vi "Launch Standard Configuration Editor.vi"   [LabVIEW 2013]
uses:
  Standard Editor/Standard Editor.lvlib
types:
  T1 = enum32{"Invalid", "Standard", "Closed", "Hidden", "Minimized", "Maximized"}
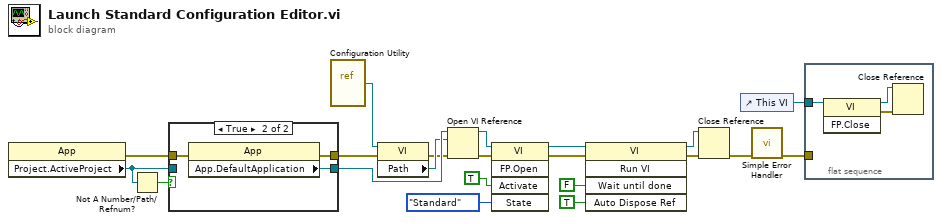
[diagram p0: block diagram]
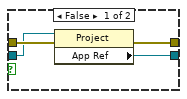
[diagram p2: hidden frame]
diagram:
  n1 = property class="App"() -> (error out=w20:errorcluster, "Project.ActiveProject"=w11:refnum<vi>)  [unwired: 2 in, 1 out]
  n2 = Not A Number/Path/Refnum?(number/path/refnum=w11) -> (NaN/Path/Refnum?=w10:bool)
  n3 = case shown="True" w10 {
    tunnel: w20 -> [w25 w28]
    tunnel: [w24 w26] -> w19
    tunnel: [w23 w27] -> w8
    tunnel: w11 -> [w22 _]
    frame False {
      n4 = property class="Project"(reference=w22, error in=w25) -> (error out=w23:errorcluster, "App Ref"=w24:refnum<vi>)  [unwired: 1 out]
    }
    frame True {
      n5 = property class="App"(error in=w28) -> (error out=w27:errorcluster, "App.DefaultApplication"=w26:refnum<vi>)  [unwired: 1 in, 1 out]
    }
  }
  n6 = vi-ref "Configuration Utility.vi"() -> (w21:refnum<vi>)
  n7 = property class="VI"(reference=w21, error in=w8) -> (error out=w17:errorcluster, "Path"=w18:path)  [unwired: 1 out]
  n8 = Open VI Reference(application reference (local)=w19, vi path=w18, error in (no error)=w17) -> (vi reference=w15:refnum<vi>, error out=w16:errorcluster)  [unwired: 3 in]
  n9 = invoke class="VI" method="FP.Open"(reference=w15, error in=w16, "Activate"=TRUE ("Activate?"), "State"=T1."Standard") -> (reference out=w6:refnum<vi>, error out=w14:errorcluster)  [unwired: 1 in, 3 out]
  n10 = invoke class="VI" method="Run VI"(reference=w6, error in=w14, "Wait until done"=FALSE ("Wait Until Done"), "Auto Dispose Ref"=TRUE ("Auto Dispose Reference")) -> (reference out=w5:refnum<vi>, error out=w7:errorcluster)  [unwired: 1 in, 3 out]
  n11 = Close Reference(reference=w5, error in (no error)=w7) -> (error out=w9:errorcluster)
  n12 = control-ref of="This VI"() -> (w3:refnum<vi>)
  n13 = call <vilib>:"Simple Error Handler.vi"("error in (no error)"=w9) -> ("error out"=w4:errorcluster)  [unwired: 4 in, 4 out]
  n14 = flat-sequence {
    tunnel: w4 -> [_]
    tunnel: w3 -> [w29]
    frame #0 {
      n15 = invoke class="VI" method="FP.Close"(reference=w29) -> (reference out=w30:refnum<vi>, error out=w31:errorcluster)  [unwired: 2 in, 1 out]
      n16 = Close Reference(reference=w30, error in (no error)=w31) -> ()  [unwired: 1 out]
    }
  }
